vi "Set Target.vi"(8 "error in (no error)":errorcluster, 9 "Target Rate (T/min)":dbl, 10 "Target Field (T)":dbl, 11 "Instrument.1820 in":refnum<class "Instrument.Oxford1820.lvclass">) -> (0 "error out":errorcluster, 2 "Response":string, 3 "Instrument.1820 in":refnum<class "Instrument.Oxford1820.lvclass">)   [LabVIEW 2019, in "Instrument.Oxford1820.lvclass"]
uses:
  Instrument.Oxford1820.lvclass
  C:/Program Files (x86)/National Instruments/LabVIEW 2019/user.lib/LevyLab/Instrument Framework/SMOs/Instrument/Instrument.lvclass
  Typedefs/PrivateEvents--Instrument.Oxford1820.setMagnetField.ctl
  <userlib>/LevyLab/Instrument Framework/Instrument Types/Cryostat/Typedefs/Magnet Axis--Enum.ctl
  <userlib>/LevyLab/Instrument Framework/Instrument Types/Cryostat/Typedefs/Magnet Mode--Enum.ctl
  <userlib>/LevyLab/Instrument Framework/SMOs/Instrument/Instrument.lvclass/Instrument.ctl
  74e6600b-75c6-4016-a9fa-b6ba76c300cd.vi
  74e6600b-75c6-4016-a9fa-b6ba76c300cd.vi/19bb5bfb-2939-4526-8ed9-dfb32c775851.vi
  74e6600b-75c6-4016-a9fa-b6ba76c300cd.vi/dd353d8c-03d3-4d07-b40c-96ac4ea50dbb.vi
  74e6600b-75c6-4016-a9fa-b6ba76c300cd.vi/19bb5bfb-2939-4526-8ed9-dfb32c775851.vi/c2c03f05-5cc9-4dc9-a4a7-aafce29be330.vi
  <userlib>/LevyLab/Instrument Framework/SMOs/Instrument/API/Send and Receive.vi
  74e6600b-75c6-4016-a9fa-b6ba76c300cd.vi/19bb5bfb-2939-4526-8ed9-dfb32c775851.vi/5187bbfd-2e35-472f-9262-5cfc4a8f7d8f.vi
  <userlib>/LevyLab/Instrument Framework/SMOs/Instrument/Private/Get Client Type.vi
  74e6600b-75c6-4016-a9fa-b6ba76c300cd.vi/dd353d8c-03d3-4d07-b40c-96ac4ea50dbb.vi/298f6b22-19d1-40f3-b8a8-333f5c265818.vi
  74e6600b-75c6-4016-a9fa-b6ba76c300cd.vi/dd353d8c-03d3-4d07-b40c-96ac4ea50dbb.vi/c421bc0d-39cf-4993-86cd-30de00834a05.vi
  74e6600b-75c6-4016-a9fa-b6ba76c300cd.vi/19bb5bfb-2939-4526-8ed9-dfb32c775851.vi/c2c03f05-5cc9-4dc9-a4a7-aafce29be330.vi/3a6d8467-c0de-41cf-9bc6-0162e6714db1.vi
  74e6600b-75c6-4016-a9fa-b6ba76c300cd.vi/19bb5bfb-2939-4526-8ed9-dfb32c775851.vi/c2c03f05-5cc9-4dc9-a4a7-aafce29be330.vi/475c7ccc-bd86-42c2-bb32-cc518c961fef.vi
  74e6600b-75c6-4016-a9fa-b6ba76c300cd.vi/19bb5bfb-2939-4526-8ed9-dfb32c775851.vi/5187bbfd-2e35-472f-9262-5cfc4a8f7d8f.vi/86ad3406-a340-41e2-a2e4-4ee2f8cad219.vi
  74e6600b-75c6-4016-a9fa-b6ba76c300cd.vi/19bb5bfb-2939-4526-8ed9-dfb32c775851.vi/5187bbfd-2e35-472f-9262-5cfc4a8f7d8f.vi/7b4e8717-018e-4a22-8f99-f698a2b71b4f.vi
  74e6600b-75c6-4016-a9fa-b6ba76c300cd.vi/19bb5bfb-2939-4526-8ed9-dfb32c775851.vi/5187bbfd-2e35-472f-9262-5cfc4a8f7d8f.vi/86ad3406-a340-41e2-a2e4-4ee2f8cad219.vi/ed650245-8b9b-424b-b4f7-11894cd4a7ea.vi
  74e6600b-75c6-4016-a9fa-b6ba76c300cd.vi/19bb5bfb-2939-4526-8ed9-dfb32c775851.vi/5187bbfd-2e35-472f-9262-5cfc4a8f7d8f.vi/86ad3406-a340-41e2-a2e4-4ee2f8cad219.vi/fc591c59-573e-470a-a57b-0ada7d995e49.vi
  <userlib>/LevyLab/Instrument Framework/SMOs/Instrument/Private/Get RC Connection Status.vi
  <userlib>/LevyLab/Instrument Framework/SMOs/Instrument/API/Enum to String.vi
  <userlib>/LevyLab/Instrument Framework/SMOs/RemoteControl/API/Send and Receive.vi
  <vilib>/Utility/Data Type/Get Type Information.vi
  <vilib>/JDP Science/JSONtext/JSON text to Variant.vi
  <userlib>/LevyLab/Instrument Framework/SMOs/Instrument/API/Instrument.GetPublicEvents.vi
  <vilib>/JDP Science/JSONtext/Variant to JSON Text.vi
  <vilib>/National Instruments/GUID Generator/Guid Generator.vi
  <userlib>/LevyLab/Instrument Framework/SMOs/Instrument/API/Instrument.MessageToProcess.vi
  <userlib>/LevyLab/Instrument Framework/SMOs/Instrument/Private/Instrument.MessageFromProcess.EventStructure.vi
  <vilib>/JDP Science/JSONtext/LVClass Serializer/JSONtext LVClass Serializer.lvclass
  <userlib>/LevyLab/Instrument Framework/Instrument Types/Cryostat/Instrument.Cryostat.lvclass
  Typedefs/Instrument.Oxford1820.protectedCommands-enum.ctl
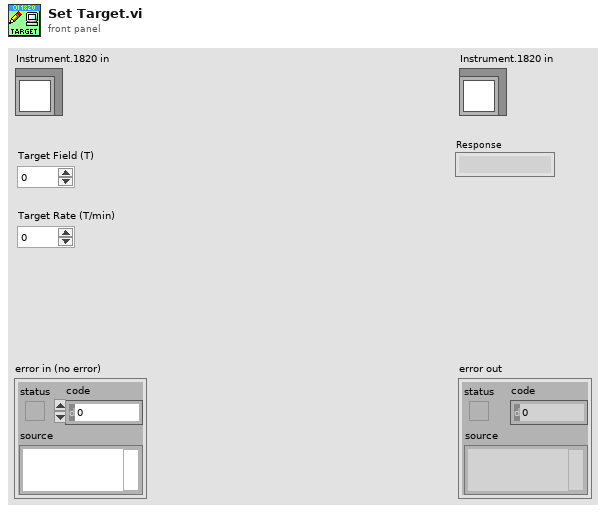
[diagram p1: front panel]
types:
  T1 = typedef "Instrument.Oxford1820.lvclass/Instrument.Oxford1820.protectedCommands-enum.ctl" = enum16{"setAction", "setTarget", "setSwitchHeat", "setLambda", "setFillMode", "setNeedleValve", "getStatus", "getTarget", "getSwitchHeat", "getPSUField", "setSequenceStatus"}
  T2 = typedef "Instrument.Oxford1820.lvclass/PrivateEvents--Instrument.Oxford1820.setMagnetField.ctl" = cluster{"field":dbl, "rate":dbl, "axis":T3, "mode":T4}
  T3 = typedef "Instrument.Cryostat.lvclass/Magnet Axis--Enum.ctl" = enum16{"Z", "X", "Y"}
  T4 = typedef "Instrument.Cryostat.lvclass/Magnet Mode--Enum.ctl" = enum16{"Persistent", "Driven"}
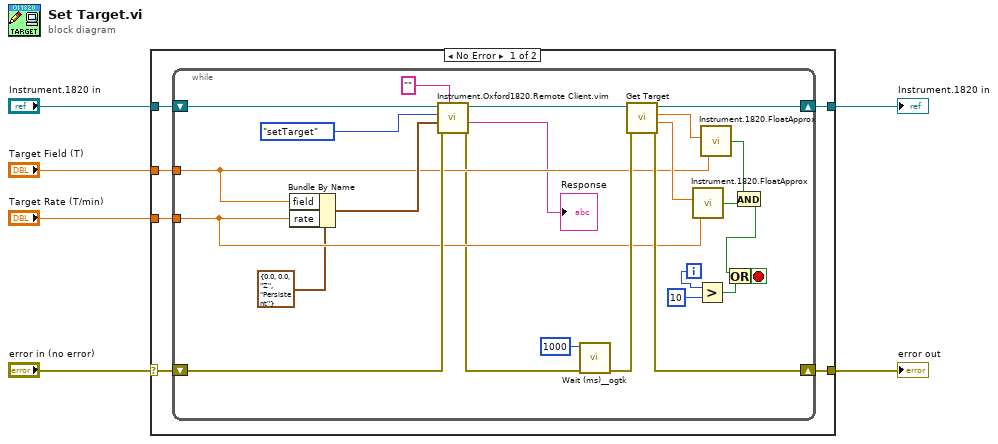
[diagram p0: block diagram]
diagram:
  n1 = case shown="No Error" "error in (no error)" {
    selector: "error in (no error)" -> [w9 w38]
    tunnel: "Target Rate (T/min)" -> [w12 _]
    tunnel: [w7 w38] -> w5
    tunnel: "Target Field (T)" -> [w11 _]
    tunnel: "Instrument.1820 in" -> [w10 w37]
    tunnel: [w8 w37] -> w1
    frame No Error {
      n2 = while {
        tunnel: w12 -> [w23]
        tunnel: w11 -> [w22]
        shift-right: [w34] -> w8
        shift-left: w10 -> [w29]
        shift-right: [w33] -> w7
        shift-left: w9 -> [w35]
        i -> [w25]
        stop <- w26 stop-if-true
        n3 = Bundle By Name(cluster=T2 {"field"=0.0, "rate"=0.0, "axis"=enum."Z", "mode"=enum."Persistent"} ("Set Magnet Field"), "field"=w22, "rate"=w23) -> (w36:T2)
        n4 = call "Instrument.Oxford1820.Remote Client.vim"("Data Out type"="", "error in (no error)"=w35, "Data"=w36, "Commands"=Instrument.Oxford1820.protectedCommands-enum."setTarget", "Instrument.1820 in"=w29) -> ("error out"=w17:errorcluster, "Data out"=→"Response":string, "Instrument.1820 out"=w16:refnum<class "Instrument.Oxford1820.lvclass">)  [unwired: 4 in]
        n5 = call <userlib>:"Wait (ms)__ogtk.vi"("error in (no error)"=w17, "milliseconds to wait"=u32 1000) -> ("error out"=w32:errorcluster)  [unwired: 8 in, 1 out]
        n6 = call "Get Target.vi"("error in (no error)"=w32, "Instrument.1820 in"=w16) -> ("error out"=w33:errorcluster, "Target Field Rate (T/min)"=w24:dbl, "Target Field (T)"=w30:dbl, "Instrument.1820 in"=w34:refnum<class "Instrument.Oxford1820.lvclass">)  [unwired: 6 in]
        n7 = call "Instrument.1820.FloatApprox.vi"("y"=w23, "x"=w24) -> ("x ~ y?"=w21:bool)  [unwired: 4 in]
        n8 = Greater?(x=w25, y=10) -> (0:w27:bool)
        n9 = call "Instrument.1820.FloatApprox.vi"("y"=w22, "x"=w30) -> ("x ~ y?"=w20:bool)  [unwired: 4 in]
        n10 = And(x=w20, y=w21) -> (x .and. y?=w19:bool)
        n11 = Or(x=w19, y=w27) -> (x .or. y?=w26:bool)
      }
    }
    frame Error {
    }
  }
  "Instrument.1820 in" <- w1
  "error out" <- w5
